vi "ni579x Validate Amplifier.vi"(0 "Register Bus":T1, 1 "scope":string, 5 "enable?":bool=TRUE, 11 "Error In":errorcluster) -> (4 "Register Bus (out)":T1, 6 "coerced enable":bool=TRUE, 15 "Error Out":errorcluster)   [LabVIEW 2015, in "ni579x Config v2 Host.lvlib"]
uses:
  <instrlib>/ni579x/Config/v2/Host/ni579x Config v2 Host.lvlib
  <instrlib>/_niInstr/Register Bus/v0/Host/Public/Register Bus Session.ctl
  <instrlib>/_niInstr/Register Bus/v0/Host/Private/Session Data.ctl
  <instrlib>/_niInstr/Register Bus/v0/Host/niInstr Register Bus v0 Host.lvlib
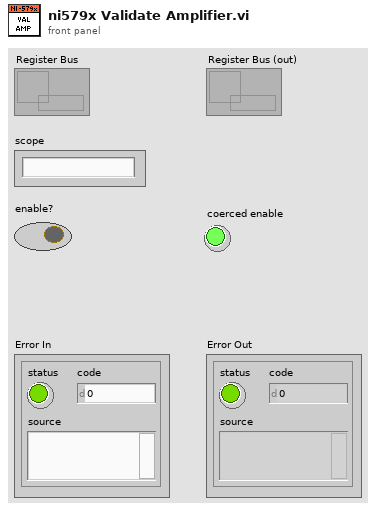
[diagram p1: front panel]
types:
  T1 = typedef "niInstr Register Bus v0 Host.lvlib/Register Bus Session.ctl" = refnum<queue>
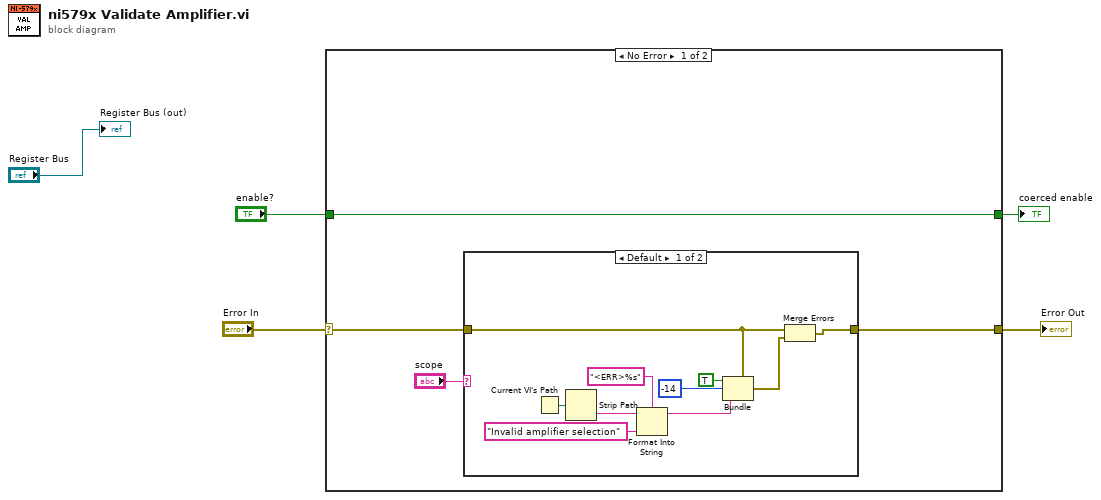
[diagram p0: block diagram]
diagram:
  n1 = case shown="No Error" "Error In" {
    selector: "Error In" -> [w7 w22]
    tunnel: [w8 w22] -> w4
    tunnel: "enable?" -> [w6 w21]
    tunnel: [w6 w21] -> w2
    frame No Error {
      n2 = case shown="Default" "scope" {
        tunnel: w7 -> [w12 w20]
        tunnel: [w10 w20] -> w8
        frame Default {
          n3 = Current VI's Path() -> (path=w14:path)
          n4 = Strip Path(path=w14) -> (name=w15:string)  [unwired: 1 out]
          n5 = Format Into String(format string="<ERR>%s", initial string=w15, "Invalid amplifier selection" ("input 1")) -> (resulting string=w16:string)  [unwired: 1 in, 1 out]
          n6 = Bundle(cluster=w12, "status"=TRUE, "code"=-14, "source"=w16) -> (w11:errorcluster)
          n7 = Merge Errors(w12, w11) -> (w10:errorcluster)
        }
        frame "rx", "tx" {
        }
      }
    }
    frame Error {
    }
  }
  "Error Out" <- w4
  "coerced enable" <- w2
  "Register Bus (out)" <- "Register Bus"
